vi "abort测试.vi"() -> ()   [LabVIEW 2019, in "test.lvlib"]
uses:
  SubVI/test.lvlib
  SubVI/SubVI.lvlib
  <vilib>/NI/Modbus Library/API/Master/Modbus Master.lvclass
  C:/Program Files (x86)/National Instruments/LabVIEW 2019/vi.lib/NI/Modbus Library/API/Modbus API.lvclass
  lib/QDInstrument.dll
panel:
  out "Instrument Ref Out":refnum<k24>
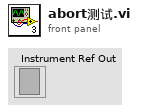
[diagram p1: front panel]
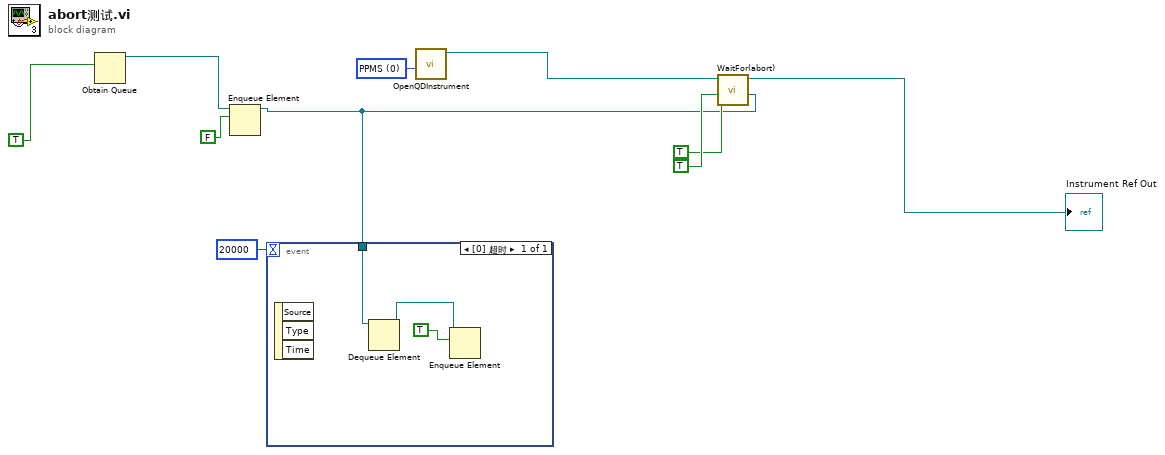
[diagram p0: block diagram]
diagram:
  w7 = 0 items=["PPMS", "VersaLab", "DynaCool", "SVSM"] ("Instrument Type")
  n1 = Obtain Queue(element data type=TRUE) -> (queue out=w3:refnum<queue>)  [unwired: 4 in, 2 out]
  n2 = Enqueue Element(queue=w3, element=FALSE ("元素")) -> (queue out=w1:refnum<queue>)  [unwired: 2 in, 2 out]
  n3 = event shown="[0] 超时" {
    selector: _ -> [_]
    dyn-events: _ -> [_]
    timeout: 20000 -> [_]
    tunnel: w1 -> [w13]
    event Timeout {
      n4 = event-data() -> ()  [unwired: 1 in, 3 out]
      n5 = Dequeue Element(queue=w13) -> (queue out=w12:refnum<queue>)  [unwired: 2 in, 3 out]
      n6 = Enqueue Element(queue=w12, element=TRUE ("元素")) -> ()  [unwired: 2 in, 3 out]
    }
  }
  n7 = call "OpenQDInstrument.vi"("Instrument Type"=w7) -> ("Instrument Ref"=w6:refnum<k24>)  [unwired: 7 in, 1 out]
  n8 = call "WaitFor(abort).vi"("config"=w1, "Wait For Field"=TRUE, "Wait For Temperature"=TRUE, "Instrument Ref In"=w6) -> ("Instrument Ref Out"=→"Instrument Ref Out":refnum<k24>)  [unwired: 6 in, 1 out]
